vi "BRig_RT__Case_Exp__State_WrongOrTimeout_Pre__v3.vi"(0 "input_dataCurrent":u16[](array[numeric]), 5 "input_WorTO":bool, 7 "input_dataBlock":u16[][](array[numeric]), 9 "input_dataTrial":u16[][](array[numeric]), 11 "input_dataExp":u16[](array[numeric])) -> (1 "output_BTPR":bool, 2 "output_T2R":bool, 3 "output_T2R_or_BTPR":u16, 4 "output_dataCurrent":u16[](array[numeric]), 8 "output_dataBlock":u16[][](array[numeric]), 10 "output_dataTrial":u16[][](array[numeric]), 12 "output_BTPRavg":dbl, 13 "output_T2Ravg":dbl, 14 "output_R(F)_or_L(T)":bool, 15 "output_haveNewAvg":bool)   [LabVIEW 2014]
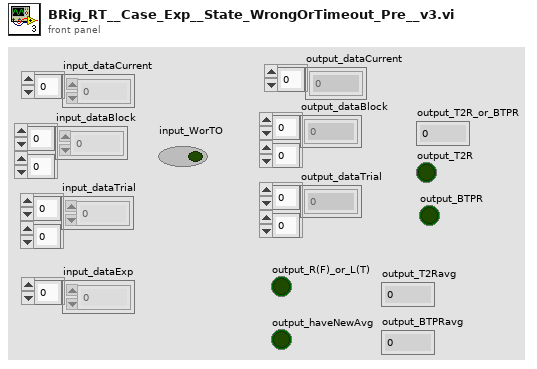
[diagram p1: front panel]
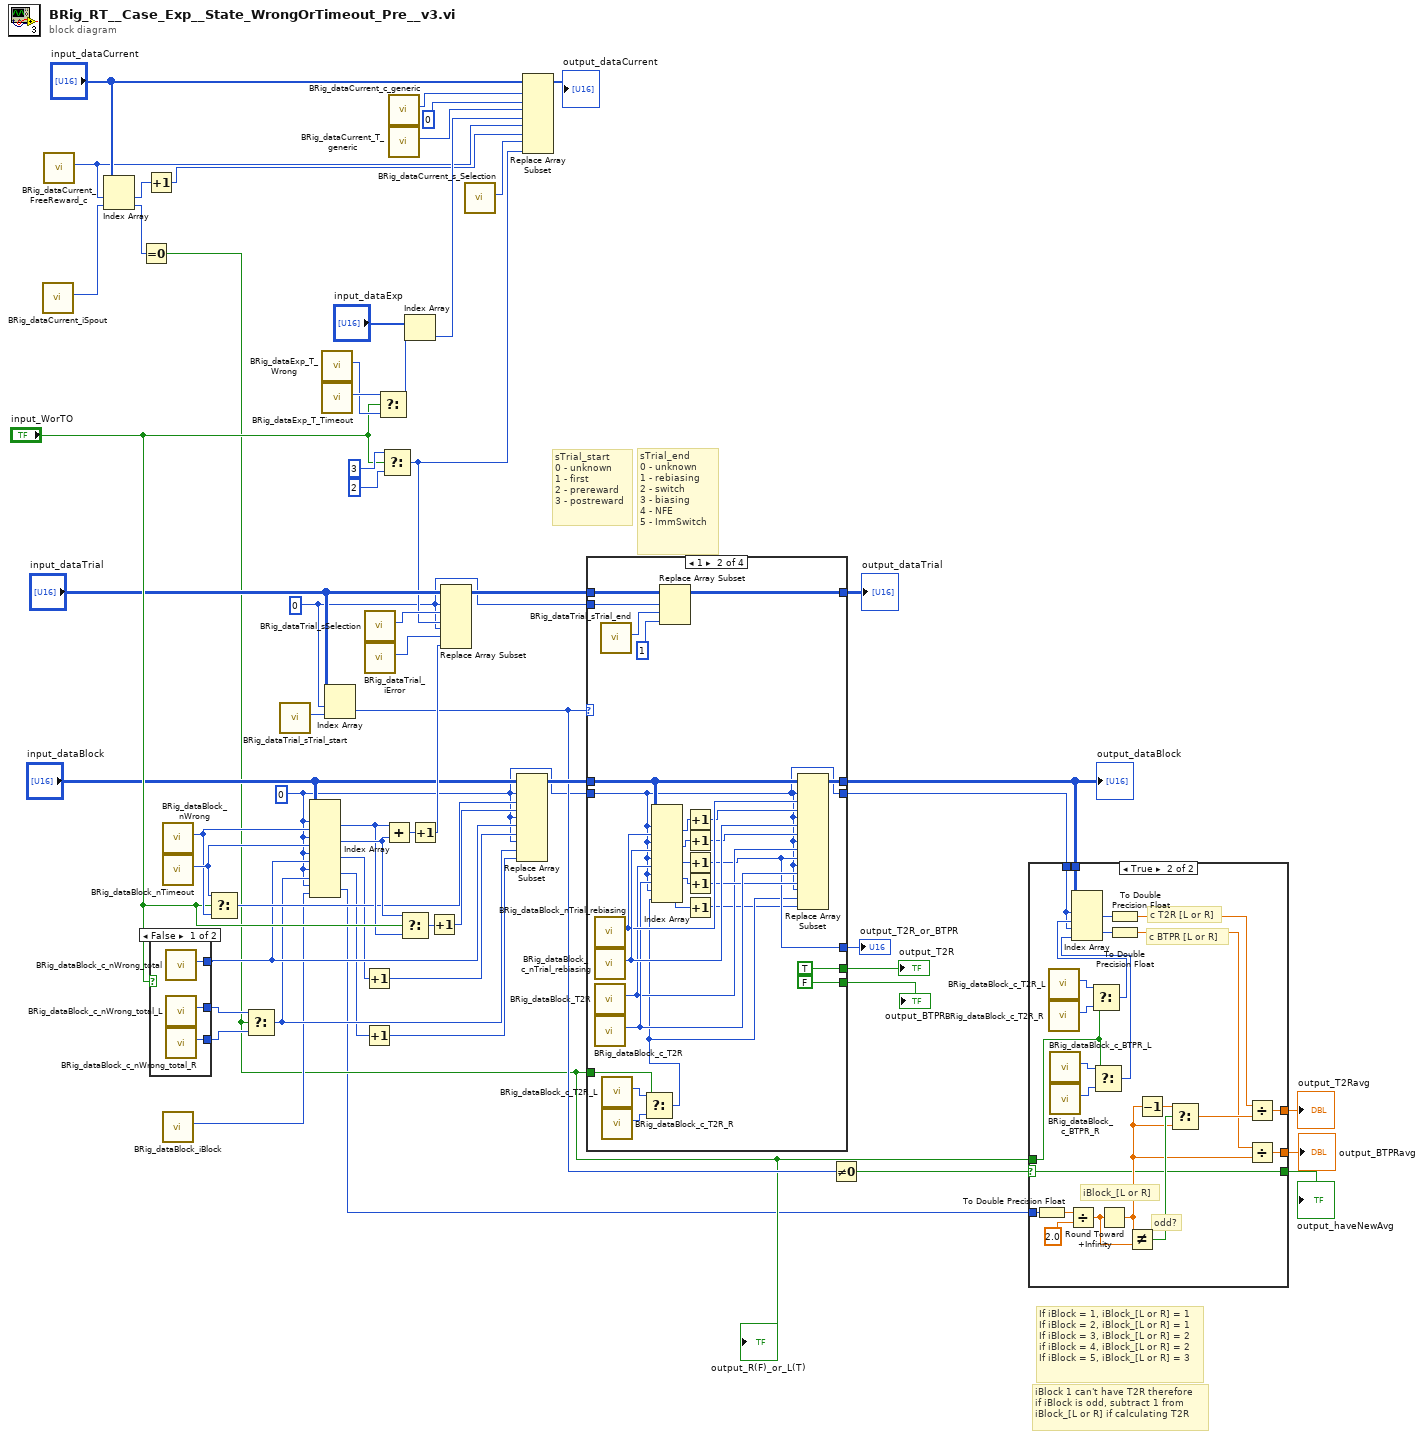
[diagram p0: block diagram]
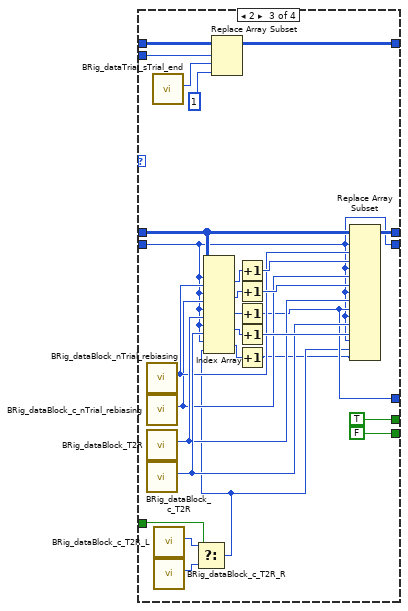
[diagram p4: hidden frame]
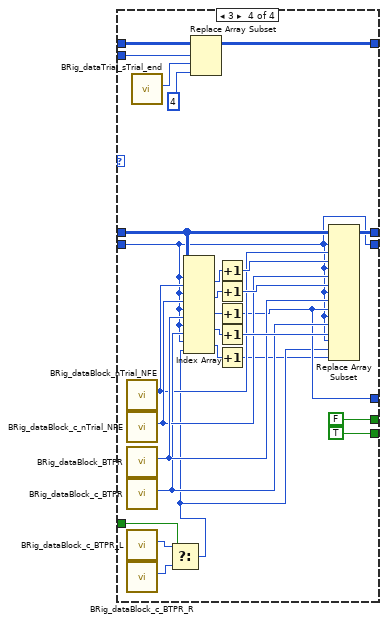
[diagram p5: hidden frame]
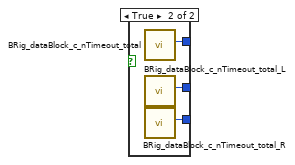
[diagram p6: hidden frame]
diagram:
  w11 = 0
  w12 = 0
  # "iBlock 1 can't have T2R therefore\nif iBlock is odd, subtract 1 from\niBlock_[L or R] if calculating T2R"
  # "If iBlock = 1, iBlock_[L or R] = 1\nIf iBlock = 2, iBlock_[L or R] = 1\nIf iBlock = 3, iBlock_[L or R] = 2\nif iBlock = 4, iBlock_[L or R] = 2\nIf iBlock = 5, iBlock_[L or R] = 3"
  # "sTrial_end\n0 - unknown\n1 - rebiasing\n2 - switch\n3 - biasing\n4 - NFE\n5 - ImmSwitch"
  # "sTrial_start\n0 - unknown\n1 - first\n2 - prereward\n3 - postreward"
  n1 = call "BRig_dataCurrent_iSpout.vi"() -> ("output_iSpout"=w10:i32)  [unwired: 11 in]
  n2 = call "BRig_dataCurrent_FreeReward_c.vi"() -> ("output_FreeReward_c"=w21:i32)  [unwired: 11 in]
  n3 = Index Array(array="input_dataCurrent", index #1=w21, index #2=w10) -> (element #1=w22:u16, element #2=w9:u16)
  n4 = Equal To 0?(x=w9) -> (x = 0?=w7:bool)
  "output_R(F)_or_L(T)" <- w7
  n5 = Increment(x=w22) -> (x+1=w20:u16)
  n6 = case shown="False" "input_WorTO" {
    tunnel: [w63 w66] -> w33
    tunnel: [w62 w65] -> w46
    tunnel: [w61 w64] -> w45
    frame False {
      n7 = call "BRig_dataBlock_c_nWrong_total.vi"() -> ("output_c_nWrong_total"=w63:i32)  [unwired: 11 in]
      n8 = call "BRig_dataBlock_c_nWrong_total_L.vi"() -> ("output_c_nWrong_total_L"=w62:i32)  [unwired: 11 in]
      n9 = call "BRig_dataBlock_c_nWrong_total_R.vi"() -> ("output_c_nWrong_total_R"=w61:i32)  [unwired: 11 in]
    }
    frame True {
      n10 = call "BRig_dataBlock_c_nTimeout_total.vi"() -> ("output_c_nTimeout_total"=w66:i32)  [unwired: 11 in]
      n11 = call "BRig_dataBlock_c_nTimeout_total_L.vi"() -> ("output_c_nTimeout_total_L"=w65:i32)  [unwired: 11 in]
      n12 = call "BRig_dataBlock_c_nTimeout_total_R.vi"() -> ("output_c_nTimeout_total_R"=w64:i32)  [unwired: 11 in]
    }
  }
  n13 = call "BRig_dataBlock_nWrong.vi"() -> ("output_nWrong"=w41:i32)  [unwired: 11 in]
  n14 = call "BRig_dataBlock_nTimeout.vi"() -> ("output_nTimeout"=w42:i32)  [unwired: 11 in]
  n15 = call "BRig_dataBlock_iBlock.vi"() -> ("output_iBlock"=w14:i32)  [unwired: 11 in]
  n16 = Select(t=w42, s="input_WorTO", f=w41) -> (s? t:f=w35:i32)
  n17 = Select(t=w46, s=w7, f=w45) -> (s? t:f=w32:i32)
  n18 = call "BRig_dataTrial_sTrial_start.vi"() -> ("output_sTrial_start"=w27:i32)  [unwired: 11 in]
  n19 = Index Array(array="input_dataBlock", index (row) #1=w11, index (col) #1=w41, index (row) #2=w11, index (col) #2=w42, index (row) #3=w11, index (col) #3=w33, index (row) #4=w11, index (col) #4=w32, index (row) #5=w11, index (col) #5=w14) -> (element #1=w38:u16, element #2=w39:u16, element #3=w31:u16, element #4=w30:u16, element #5=w4:u16)
  n20 = call "BRig_dataExp_T_Wrong.vi"() -> ("output_T_Wrong"=w52:i32)  [unwired: 11 in]
  n21 = call "BRig_dataExp_T_Timeout.vi"() -> ("output_T_Timeout"=w53:i32)  [unwired: 11 in]
  n22 = Index Array(array="input_dataTrial", index (row)=w12, index (col)=w27) -> (element=w13:u16)
  n23 = Increment(x=w31) -> (x+1=w29:u16)
  n24 = Increment(x=w30) -> (x+1=w28:u16)
  n25 = call "BRig_dataTrial_sSelection.vi"() -> ("output_sSelection"=w48:i32)  [unwired: 11 in]
  n26 = call "BRig_dataTrial_iError.vi"() -> ("output_iError"=w47:i32)  [unwired: 11 in]
  n27 = Select(t=w53, s="input_WorTO", f=w52) -> (s? t:f=w54:i32)
  n28 = Select(t=u16 3 ("new element/subarray"), s="input_WorTO", f=u16 2 ("new element/subarray")) -> (s? t:f=w18:u16)
  n29 = Add(x=w38, y=w39) -> (x+y=w44:u16)
  n30 = call "BRig_dataCurrent_c_generic.vi"() -> ("output_count_generic"=w59:i32)  [unwired: 11 in]
  n31 = call "BRig_dataCurrent_T_generic.vi"() -> ("output_T_generic"=w58:i32)  [unwired: 11 in]
  n32 = Select(t=w39, s="input_WorTO", f=w38) -> (s? t:f=w37:u16)
  n33 = Index Array(array="input_dataExp", index=w54) -> (element=w51:u16)
  n34 = Increment(x=w44) -> (x+1=w43:u16)
  n35 = Increment(x=w37) -> (x+1=w34:u16)
  n36 = Replace Array Subset(array="input_dataTrial", new element #1=w18, index (row) #1=w12, index (col) #1=w48, new element #2=w43, index (row) #2=w12, index (col) #2=w47) -> (w25:u16[][])
  n37 = call "BRig_dataCurrent_s_Selection.vi"() -> ("output_s_Selection"=w19:i32)  [unwired: 11 in]
  n38 = Replace Array Subset(array="input_dataBlock", new element #1=w34, index (row) #1=w11, index (col) #1=w35, new element #2=w29, index (row) #2=w11, index (col) #2=w33, new element #3=w28, index (row) #3=w11, index (col) #3=w32) -> (w24:u16[][])
  n39 = Replace Array Subset(array="input_dataCurrent", new element #1=u16 0 ("new element/subarray"), index #1=w59, new element #2=w51, index #2=w58, new element #3=w20, index #3=w21, new element #4=w18, index #4=w19) -> (→"output_dataCurrent":u16[])
  n40 = case shown="1" w13 {
    tunnel: w25 -> [w69 w97 w125 w153]
    tunnel: w12 -> [_ w95 w123 w151]
    tunnel: [w69 w96 w124 w152] -> w23
    tunnel: w24 -> [w68 w86 w109 w141]
    tunnel: [w68 w85 w108 w140] -> w6
    tunnel: w11 -> [w67 w70 w98 w126]
    tunnel: [_ w77 w107 w133] -> w17
    tunnel: [_ TRUE TRUE FALSE] -> w16
    tunnel: [_ FALSE FALSE TRUE] -> w15
    tunnel: w7 -> [_ w76 w100 w132]
    tunnel: [w67 w70 w98 w126] -> w5
    frame 0, Default {
    }
    frame 1 {
      n41 = call "BRig_dataBlock_nTrial_rebiasing.vi"() -> ("output_nTrial_rebiasing"=w91:i32)  [unwired: 11 in]
      n42 = call "BRig_dataBlock_c_nTrial_rebiasing.vi"() -> ("output_c_nTrial_rebiasing"=w92:i32)  [unwired: 11 in]
      n43 = call "BRig_dataBlock_T2R.vi"() -> ("output_T2R"=w80:i32)  [unwired: 11 in]
      n44 = call "BRig_dataBlock_c_T2R.vi"() -> ("output_c_T2R"=w82:i32)  [unwired: 11 in]
      n45 = call "BRig_dataTrial_sTrial_end.vi"() -> ("output_sTrial_end"=w94:i32)  [unwired: 11 in]
      n46 = call "BRig_dataBlock_c_T2R_L.vi"() -> ("output_c_T2R_L"=w75:i32)  [unwired: 11 in]
      n47 = call "BRig_dataBlock_c_T2R_R.vi"() -> ("output_c_T2R_R"=w74:i32)  [unwired: 11 in]
      n48 = Select(t=w75, s=w76, f=w74) -> (s? t:f=w72:i32)
      n49 = Index Array(array=w86, index (row) #1=w70, index (col) #1=w91, index (row) #2=w70, index (col) #2=w92, index (row) #3=w70, index (col) #3=w80, index (row) #4=w70, index (col) #4=w82, index (row) #5=w70, index (col) #5=w72) -> (element #1=w90:u16, element #2=w88:u16, element #3=w84:u16, element #4=w83:u16, element #5=w73:u16)
      n50 = Replace Array Subset(array=w97, new element=u16 1 ("new element/subarray"), index (row)=w95, index (col)=w94) -> (w96:u16[][])
      n51 = Increment(x=w90) -> (x+1=w89:u16)
      n52 = Increment(x=w88) -> (x+1=w87:u16)
      n53 = Increment(x=w84) -> (x+1=w77:u16)
      n54 = Increment(x=w83) -> (x+1=w81:u16)
      n55 = Increment(x=w73) -> (x+1=w71:u16)
      n56 = Replace Array Subset(array=w86, new element #1=w89, index (row) #1=w70, index (col) #1=w91, new element #2=w87, index (row) #2=w70, index (col) #2=w92, new element #3=w77, index (row) #3=w70, index (col) #3=w80, new element #4=w81, index (row) #4=w70, index (col) #4=w82, new element #5=w71, index (row) #5=w70, index (col) #5=w72) -> (w85:u16[][])
    }
    frame 2 {
      n57 = call "BRig_dataBlock_nTrial_rebiasing.vi"() -> ("output_nTrial_rebiasing"=w111:i32)  [unwired: 11 in]
      n58 = call "BRig_dataBlock_c_nTrial_rebiasing.vi"() -> ("output_c_nTrial_rebiasing"=w110:i32)  [unwired: 11 in]
      n59 = call "BRig_dataBlock_T2R.vi"() -> ("output_T2R"=w118:i32)  [unwired: 11 in]
      n60 = call "BRig_dataBlock_c_T2R.vi"() -> ("output_c_T2R"=w119:i32)  [unwired: 11 in]
      n61 = call "BRig_dataTrial_sTrial_end.vi"() -> ("output_sTrial_end"=w122:i32)  [unwired: 11 in]
      n62 = call "BRig_dataBlock_c_T2R_L.vi"() -> ("output_c_T2R_L"=w104:i32)  [unwired: 11 in]
      n63 = call "BRig_dataBlock_c_T2R_R.vi"() -> ("output_c_T2R_R"=w103:i32)  [unwired: 11 in]
      n64 = Select(t=w104, s=w100, f=w103) -> (s? t:f=w101:i32)
      n65 = Index Array(array=w109, index (row) #1=w98, index (col) #1=w111, index (row) #2=w98, index (col) #2=w110, index (row) #3=w98, index (col) #3=w118, index (row) #4=w98, index (col) #4=w119, index (row) #5=w98, index (col) #5=w101) -> (element #1=w112:u16, element #2=w114:u16, element #3=w116:u16, element #4=w117:u16, element #5=w102:u16)
      n66 = Replace Array Subset(array=w125, new element=u16 1 ("new element/subarray"), index (row)=w123, index (col)=w122) -> (w124:u16[][])
      n67 = Increment(x=w112) -> (x+1=w113:u16)
      n68 = Increment(x=w114) -> (x+1=w115:u16)
      n69 = Increment(x=w116) -> (x+1=w107:u16)
      n70 = Increment(x=w117) -> (x+1=w120:u16)
      n71 = Increment(x=w102) -> (x+1=w99:u16)
      n72 = Replace Array Subset(array=w109, new element #1=w113, index (row) #1=w98, index (col) #1=w111, new element #2=w115, index (row) #2=w98, index (col) #2=w110, new element #3=w107, index (row) #3=w98, index (col) #3=w118, new element #4=w120, index (row) #4=w98, index (col) #4=w119, new element #5=w99, index (row) #5=w98, index (col) #5=w101) -> (w108:u16[][])
    }
    frame 3 {
      n73 = call "BRig_dataBlock_nTrial_NFE.vi"() -> ("output_nTrial_NFE"=w136:i32)  [unwired: 11 in]
      n74 = call "BRig_dataBlock_c_nTrial_NFE.vi"() -> ("output_c_nTrial_NFE"=w138:i32)  [unwired: 11 in]
      n75 = call "BRig_dataBlock_BTPR.vi"() -> ("output_BTPR"=w139:i32)  [unwired: 11 in]
      n76 = call "BRig_dataBlock_c_BTPR.vi"() -> ("output_c_BTPR"=w137:i32)  [unwired: 11 in]
      n77 = call "BRig_dataBlock_c_BTPR_L.vi"() -> ("output_c_BTPR_L"=w131:i32)  [unwired: 11 in]
      n78 = call "BRig_dataBlock_c_BTPR_R.vi"() -> ("output_c_BTPR_R"=w130:i32)  [unwired: 11 in]
      n79 = call "BRig_dataTrial_sTrial_end.vi"() -> ("output_sTrial_end"=w150:i32)  [unwired: 11 in]
      n80 = Select(t=w131, s=w132, f=w130) -> (s? t:f=w128:i32)
      n81 = Index Array(array=w141, index (row) #1=w126, index (col) #1=w136, index (row) #2=w126, index (col) #2=w138, index (row) #3=w126, index (col) #3=w139, index (row) #4=w126, index (col) #4=w137, index (row) #5=w126, index (col) #5=w128) -> (element #1=w142:u16, element #2=w144:u16, element #3=w146:u16, element #4=w147:u16, element #5=w129:u16)
      n82 = Replace Array Subset(array=w153, new element=u16 4 ("new element/subarray"), index (row)=w151, index (col)=w150) -> (w152:u16[][])
      n83 = Increment(x=w142) -> (x+1=w143:u16)
      n84 = Increment(x=w144) -> (x+1=w145:u16)
      n85 = Increment(x=w146) -> (x+1=w133:u16)
      n86 = Increment(x=w147) -> (x+1=w148:u16)
      n87 = Increment(x=w129) -> (x+1=w127:u16)
      n88 = Replace Array Subset(array=w141, new element #1=w143, index (row) #1=w126, index (col) #1=w136, new element #2=w145, index (row) #2=w126, index (col) #2=w138, new element #3=w133, index (row) #3=w126, index (col) #3=w139, new element #4=w148, index (row) #4=w126, index (col) #4=w137, new element #5=w127, index (row) #5=w126, index (col) #5=w128) -> (w140:u16[][])
    }
  }
  "output_dataBlock" <- w6
  "output_dataTrial" <- w23
  "output_T2R_or_BTPR" <- w17
  "output_T2R" <- w16
  "output_BTPR" <- w15
  n89 = Not Equal To 0?(x=w13) -> (x != 0?=w8:bool)
  n90 = case shown="True" w8 {
    selector: w8 -> [_ w154]
    tunnel: w7 -> [_ w169]
    tunnel: w6 -> [_ w172]
    tunnel: w5 -> [_ w171]
    tunnel: w4 -> [_ w165]
    tunnel: [_ w156] -> w3
    tunnel: [_ w155] -> w2
    tunnel: [_ w154] -> w1
    frame False {
    }
    frame True {
      # "c BTPR [L or R]"
      # "c T2R [L or R]"
      # "odd?"
      # "iBlock_[L or R]"
      n91 = To Double Precision Float(number=w165) -> (double precision float=w168:dbl)
      n92 = call "BRig_dataBlock_c_T2R_L.vi"() -> ("output_c_T2R_L"=w176:i32)  [unwired: 11 in]
      n93 = call "BRig_dataBlock_c_T2R_R.vi"() -> ("output_c_T2R_R"=w177:i32)  [unwired: 11 in]
      n94 = call "BRig_dataBlock_c_BTPR_L.vi"() -> ("output_c_BTPR_L"=w174:i32)  [unwired: 11 in]
      n95 = call "BRig_dataBlock_c_BTPR_R.vi"() -> ("output_c_BTPR_R"=w175:i32)  [unwired: 11 in]
      n96 = Divide(x=w168, y=2.0) -> (x/y=w166:dbl)
      n97 = Select(t=w176, s=w169, f=w177) -> (s? t:f=w173:i32)
      n98 = Select(t=w174, s=w169, f=w175) -> (s? t:f=w170:i32)
      n99 = Index Array(array=w172, index (row) #1=w171, index (col) #1=w173, index (row) #2=w171, index (col) #2=w170) -> (element #1=w160:u16, element #2=w161:u16)
      n100 = Round Toward +Infinity(x=w166) -> (ceil(x): smallest int >= x=w159:dbl)
      n101 = To Double Precision Float(number=w160) -> (double precision float=w158:dbl)
      n102 = To Double Precision Float(number=w161) -> (double precision float=w157:dbl)
      n103 = Not Equal?(x=w159, y=w166) -> (x != y?=w163:bool)
      n104 = Decrement(x=w159) -> (x-1=w164:dbl)
      n105 = Select(t=w164, s=w163, f=w159) -> (s? t:f=w162:dbl)
      n106 = Divide(x=w158, y=w162) -> (x/y=w156:dbl)
      n107 = Divide(x=w157, y=w159) -> (x/y=w155:dbl)
    }
  }
  "output_T2Ravg" <- w3
  "output_BTPRavg" <- w2
  "output_haveNewAvg" <- w1
